vi "Configure Joystick Axis Target.vi"(5 "Target Axis Number (1)":u8=1, 6 "Target Axis Type (0: axis)":u16(ring) items=["axis", "lockstep group", "virtual axis"], 7 "Target Device Number (1)":u8=1, 8 "error in (no error)":errorcluster, 9 "Joystick Device Number":string, 10 "Joystick Axis Number (1)":u8=1 min=1 step=1, 11 "VISA resource name":refnum<visa-resource-name>) -> (0 "error out":errorcluster, 3 "VISA resource name out":refnum<visa-resource-name>)   [LabVIEW 2018, in "Zaber A Series.lvlib"]
doc: "Use this VI to set the target for a single joystick axis - that is, which motion device moves in response to joystick movements.\n\nSelect the device number of the joystick and which axis to configure - 1 is the horizontal axis, 2 the vertical and 3 is the rotation of the knob on the end of the stick.\n\nThe Target Device Number input is the device number that the joystick will address motion commands to when ths selected axis of the joystick is moved.\n\nThe Target Axis Number is the number of the axis, lockstep group or virtual axis to move. The Target Axis Type input controls which type of axis is targeted. \n\nThis VI expects the serial port to have already been configured."
uses:
  Zaber A Series.lvlib
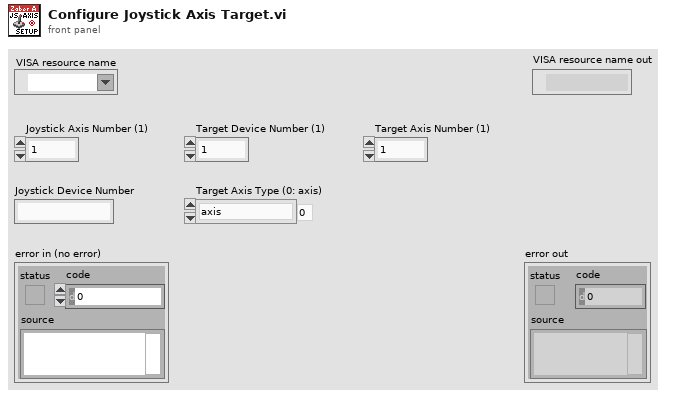
[diagram p1: front panel]
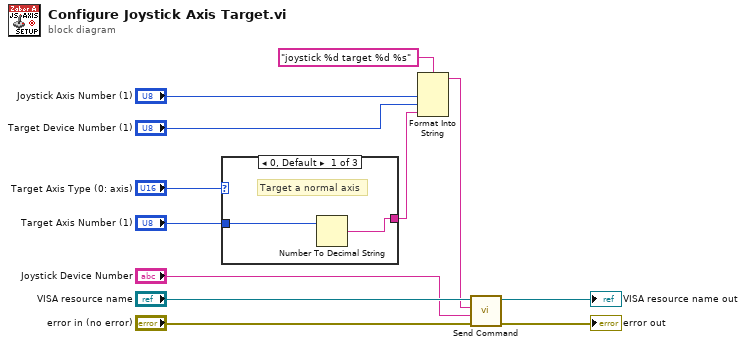
[diagram p0: block diagram]
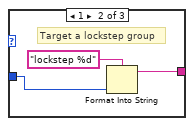
[diagram p2: hidden frame]
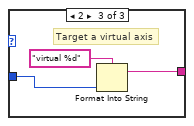
[diagram p3: hidden frame]
diagram:
  n1 = case shown="0, Default" "Target Axis Type (0: axis)" {
    tunnel: [w14 w15 w18] -> w4
    tunnel: "Target Axis Number (1)" -> [w13 w16 w19]
    frame 0, Default {
      # "Target a normal axis"
      n2 = Number To Decimal String(number=w13) -> (decimal integer string=w14:string)  [unwired: 1 in]
    }
    frame 1 {
      # "Target a lockstep group"
      n3 = Format Into String(format string="lockstep %d", w16) -> (resulting string=w15:string)  [unwired: 2 in, 1 out]
    }
    frame 2 {
      # "Target a virtual axis"
      n4 = Format Into String(format string="virtual %d", w19) -> (resulting string=w18:string)  [unwired: 2 in, 1 out]
    }
  }
  n5 = Format Into String(format string="joystick %d target %d %s", "Joystick Axis Number (1)", "Target Device Number (1)", w4) -> (resulting string=w6:string)  [unwired: 2 in, 1 out]
  n6 = call "Send Command.vi"("error in (no error)"="error in (no error)", "Device and Axis"="Joystick Device Number", "Command"=w6, "VISA resource name"="VISA resource name") -> ("error out"=→"error out":errorcluster, "VISA resource name out"=→"VISA resource name out":refnum<visa-resource-name>)  [unwired: 2 in, 4 out]
